vi "Arcade Drive.vi"(8 "Max Output":dbl, 10 "Y Axis":dbl, 11 "X Axis":dbl) -> (2 "Left Motor Value":dbl, 3 "Right Motor Value":dbl)   [LabVIEW 2012]
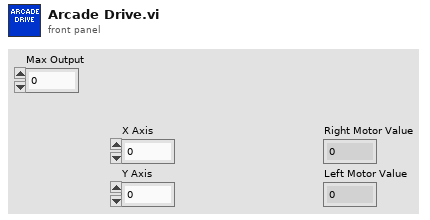
[diagram p1: front panel]
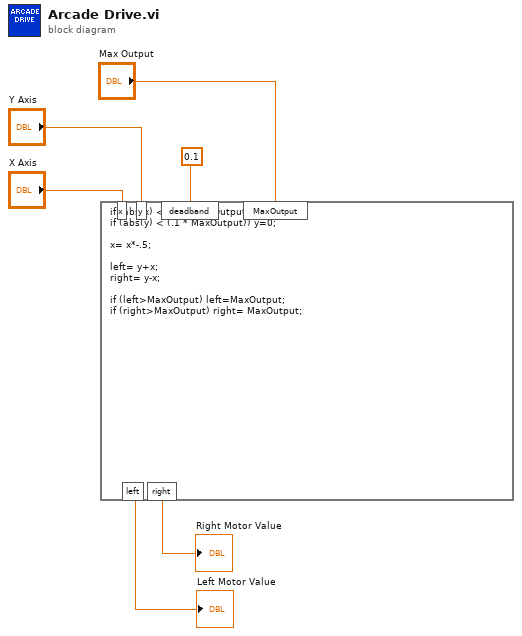
[diagram p0: block diagram]
diagram:
  n1 = formula code="if (abs(x) < (.15* MaxOutput)) x=0;\nif (abs(y) < (.1 * MaxOutput)) y=0; \n\nx= x*-.5;\n\nleft= y+x;\nright= y-x;\n\nif (left>MaxOutput) left=MaxOutput;\nif (right>MaxOutput) right= MaxOutput;"("x"="X Axis", "y"="Y Axis", "deadband"=0.1 ("input variable"), "MaxOutput"="Max Output") -> ("left"=→"Left Motor Value":dbl, "right"=→"Right Motor Value":dbl)
